vi "编辑文本.vi"(8 "error in (no error)":errorcluster caption="错误输入（无错误）", 9 "扫描代码":i16, 11 "程序响应 输入":refnum<class "程序响应.lvclass">) -> (0 "error out":errorcluster caption="错误输出", 3 "程序响应 输出":refnum<class "程序响应.lvclass">)   [LabVIEW 2020, in "程序响应.lvlib" / "程序响应.lvclass"]
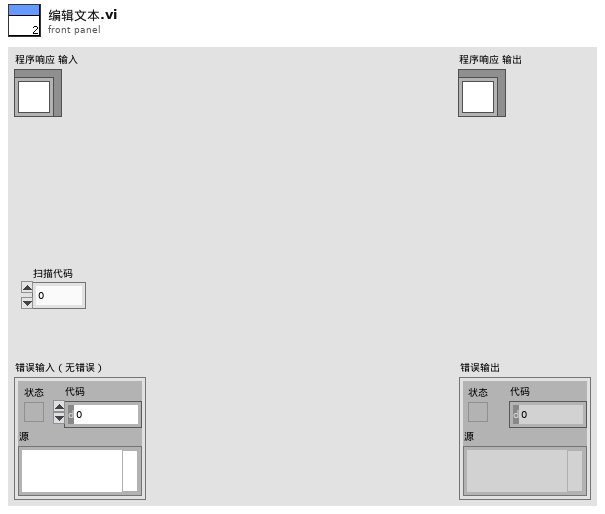
[diagram p1: front panel]
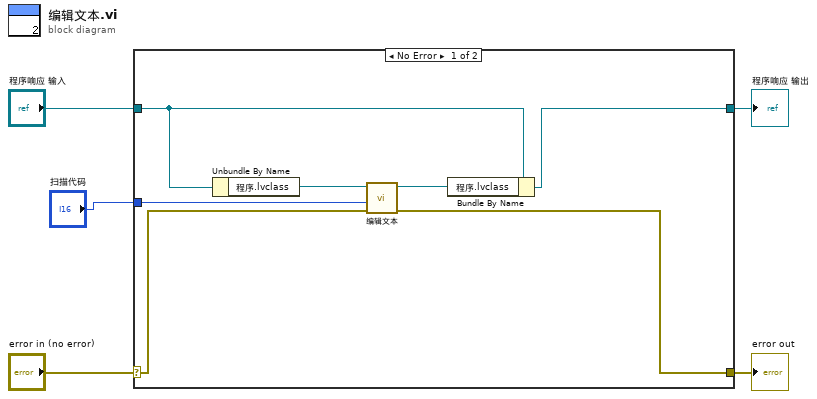
[diagram p0: block diagram]
diagram:
  n1 = case shown="No Error" "error in (no error)" {
    selector: "error in (no error)" -> [w8 w14]
    tunnel: [w7 w14] -> w4
    tunnel: [w9 w13] -> w2
    tunnel: "程序响应 输入" -> [w10 w13]
    tunnel: "扫描代码" -> [w6 _]
    frame No Error {
      n2 = Unbundle By Name(w10) -> ("程序.lvclass"=w12:refnum<class "程序.lvclass">)
      n3 = call-dynamic "编辑文本.vi"("error in (no error)"=w8, "扫描代码"=w6, "程序 输入"=w12) -> ("error out"=w7:errorcluster, "程序 输出"=w11:refnum<class "程序.lvclass">)  [unwired: 7 in]
      n4 = Bundle By Name(cluster=w10, "程序.lvclass"=w11) -> (w9:refnum<class "程序响应.lvclass">)
    }
    frame Error {
    }
  }
  "error out" <- w4
  "程序响应 输出" <- w2
